vi "To JSON Tree.vi"(8 "error in (no error)":errorcluster, 11 "Response in":refnum<class "Response.lvclass">) -> (0 "error out":errorcluster, 2 "JSON Tree Out":variant, 3 "Response out":refnum<class "Response.lvclass">)   [LabVIEW 2015, in "Response.lvclass"]
uses:
  Response.lvclass
  <vilib>/rajsite/i3-json/JSON Generation/Add Object Parameter Files/Add Object Parameter - Known Type.vi
  <vilib>/rajsite/i3-json/JSON Generation/Create Value Files/Create Value - Object.vi
  <vilib>/rajsite/i3-json/JSON Generation/Add Object Parameter Files/Add Object Parameter - String.vi
  id/id.lvclass
  JSONable/JSONable.lvclass
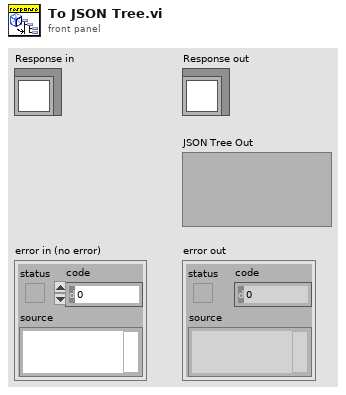
[diagram p1: front panel]
types:
  T1 = typedef "i3-json.lvlib/JSON Type.ctl" = enum8{"JSON Compatible", "JSON Array", "JSON Object", "JSON Null", "Double", "String", "Boolean", "Unknown"}
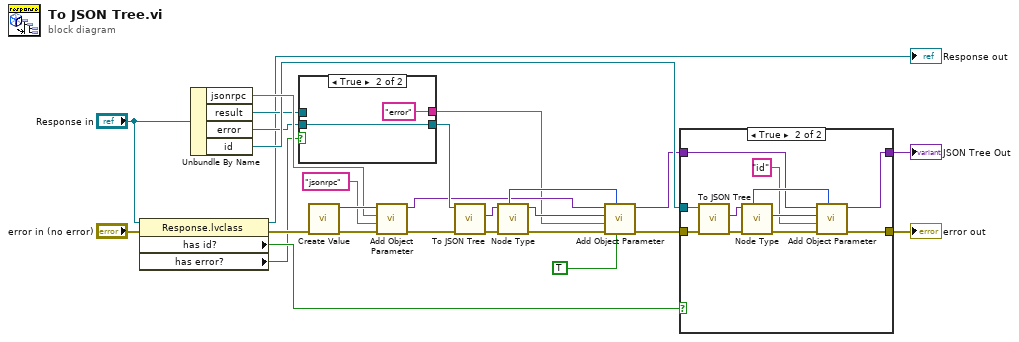
[diagram p0: block diagram]
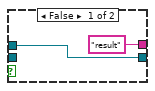
[diagram p2: hidden frame]
diagram:
  n1 = property class="Response.lvclass"(reference="Response in", error in="error in (no error)") -> (reference out=→"Response out":refnum<class "Response.lvclass">, error out=w17:errorcluster, "has id?"=w22:bool, "has error?"=w4:bool)
  n2 = Unbundle By Name("Response in") -> ("jsonrpc"=w26:string, "result"=w9:refnum<class "result.lvclass">, "error"=w8:refnum<class "error.lvclass">, "id"=w21:refnum<class "id.lvclass">)
  n3 = case shown="True" w4 {
    tunnel: w8 -> [_ w30]
    tunnel: ["result" ("f") "error"] -> w1
    tunnel: [w28 w30] -> w11
    tunnel: w9 -> [w28 _]
    frame False {
    }
    frame True {
    }
  }
  n4 = call-poly <vilib>:"Create Value.vi"("error in (no error)"=w17) -> ("error out"=w24:errorcluster, "JSON Tree"=w27:variant)  [unwired: 9 in]
  n5 = call-poly <vilib>:"Add Object Parameter.vi"("error in (no error)"=w24, "Name"="jsonrpc", "String"=w26, "JSON Tree in (JSON Object)"=w27) -> ("error out"=w2:errorcluster, "JSON Tree out (JSON Object)"=w7:variant)  [unwired: 6 in]
  n6 = call-dynamic "To JSON Tree.vi"("error in (no error)"=w2, "JSONable in"=w11) -> ("error out"=w14:errorcluster, "JSON Tree Out"=w12:variant)  [unwired: 7 in, 1 out]
  n7 = call <vilib>:"Node Type.vi"("error in (no error)"=w14, "JSON Tree In"=w12) -> ("error out"=w15:errorcluster, "JSON Tree Out"=w10:variant, "JSON Type"=w13:T1)  [unwired: 5 in, 2 out]
  n8 = call-poly <vilib>:"Add Object Parameter.vi"("Add Parameter as JSON Tree?"=TRUE, "JSON Type"=w13, "error in (no error)"=w15, "Name"=w1, "Value"=w10, "JSON Tree in (JSON Object)"=w7) -> ("error out"=w5:errorcluster, "JSON Tree out (JSON Object)"=w6:variant)  [unwired: 4 in]
  n9 = case shown="True" w22 {
    tunnel: [w32 w38] -> w19
    tunnel: [w33 w39] -> w20
    tunnel: w21 -> [_ w37]
    tunnel: w5 -> [w32 w36]
    tunnel: w6 -> [w33 w35]
    frame False {
    }
    frame True {
      n10 = call-dynamic "To JSON Tree.vi"("error in (no error)"=w36, "id in"=w37) -> ("error out"=w41:errorcluster, "JSON Tree Out"=w44:variant)  [unwired: 7 in, 1 out]
      n11 = call <vilib>:"Node Type.vi"("error in (no error)"=w41, "JSON Tree In"=w44) -> ("error out"=w40:errorcluster, "Value"=w42:variant, "JSON Type"=w43:T1)  [unwired: 5 in, 2 out]
      n12 = call-poly <vilib>:"Add Object Parameter.vi"("JSON Type"=w43, "error in (no error)"=w40, "Name"="id", "Value"=w42, "JSON Tree in (JSON Object)"=w35) -> ("error out"=w38:errorcluster, "JSON Tree out (JSON Object)"=w39:variant)  [unwired: 5 in]
    }
  }
  "error out" <- w19
  "JSON Tree Out" <- w20
